vi "Setting.vi"() -> ()   [LabVIEW 2020]
uses:
  Libraries/S7/S7.lvlib
  Global_Variable/Global.vi
  <userlib>/_MGI/1D Array/MGI Average/MGI Average (DBL[]).vi
panel:
  in  "速度":sgl format="%#_3f RMP"
  out "退出":bool=TRUE
  in  "STEP":string
  in  "工位二标定":bool
  in  "停止":bool
  in  "工位一标定":bool
  out "标定曲线":cluster{dbl[], dbl[]}[](graph)
  # "配置标定"
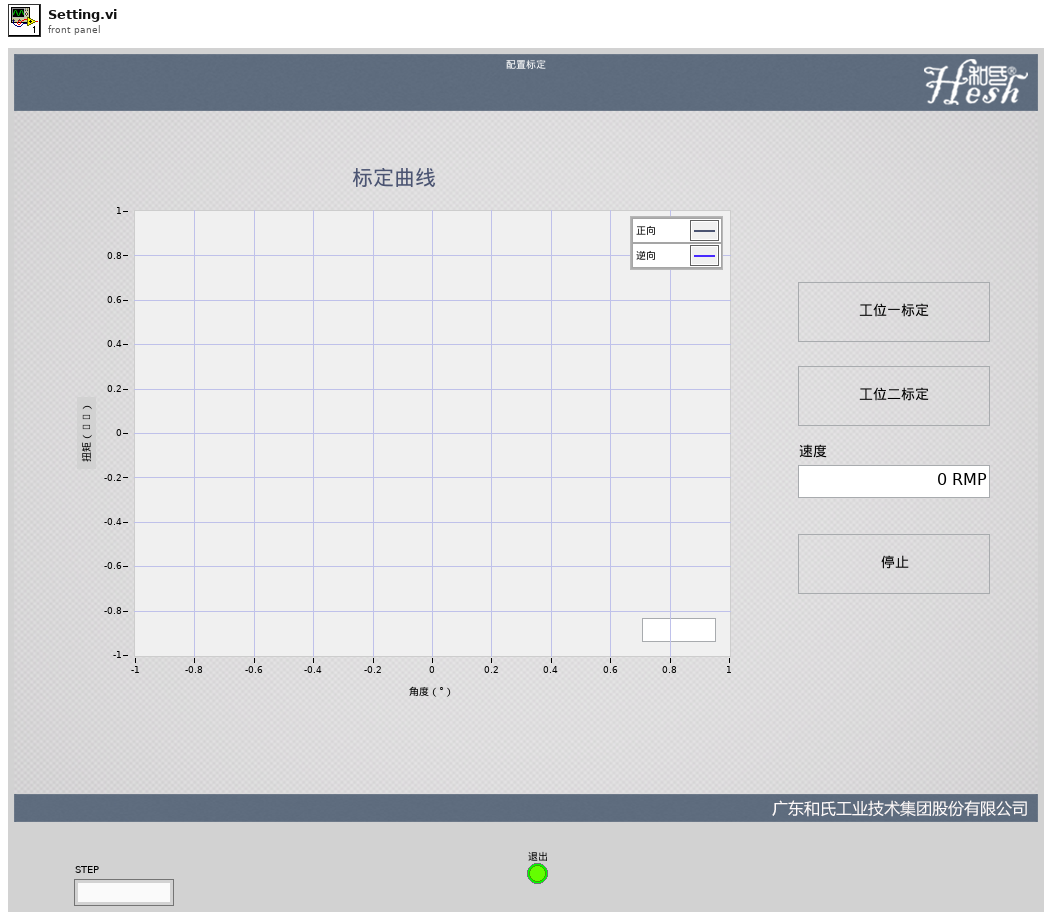
[diagram p1: front panel]
types:
  T1 = cluster{"左工位驱动伺服位移":sgl, "右工位驱动伺服位移":sgl, "横向伺服位移":sgl, "左加载伺服位移":sgl, "右加载伺服位移":sgl}
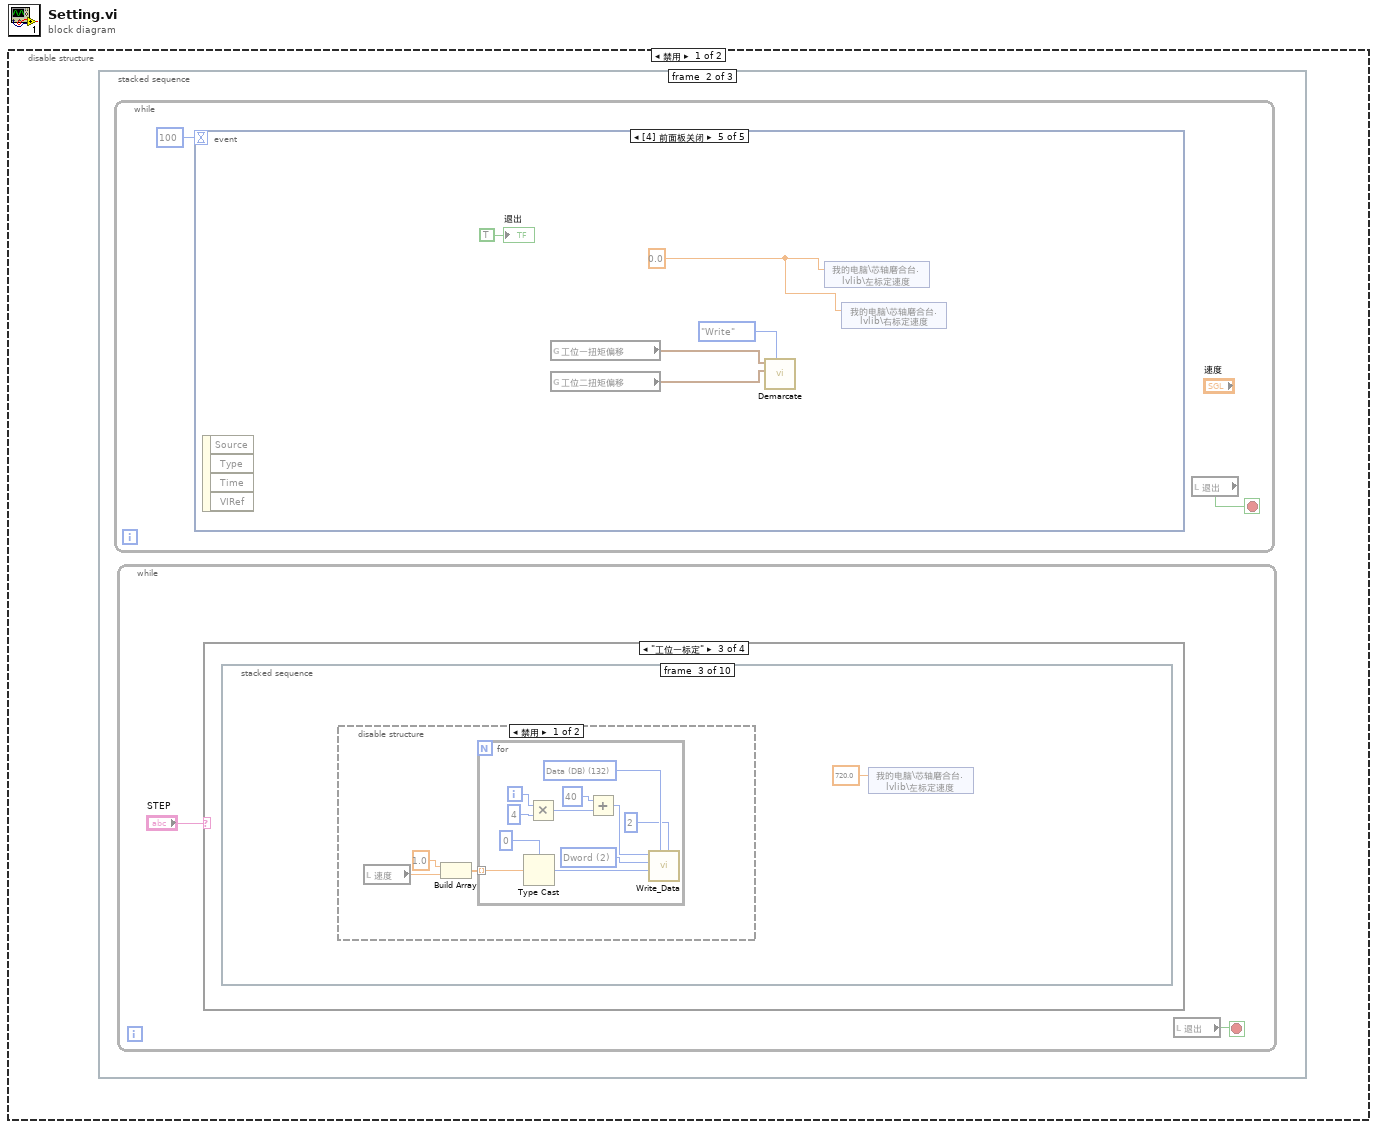
[diagram p0: block diagram]
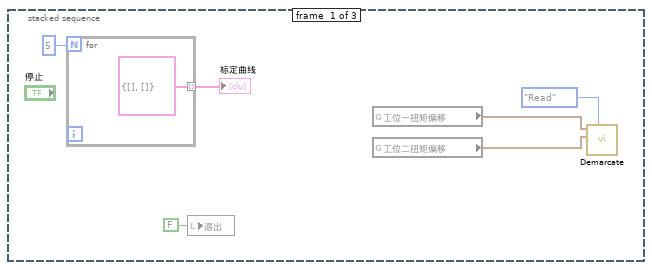
[diagram p2: hidden frame]
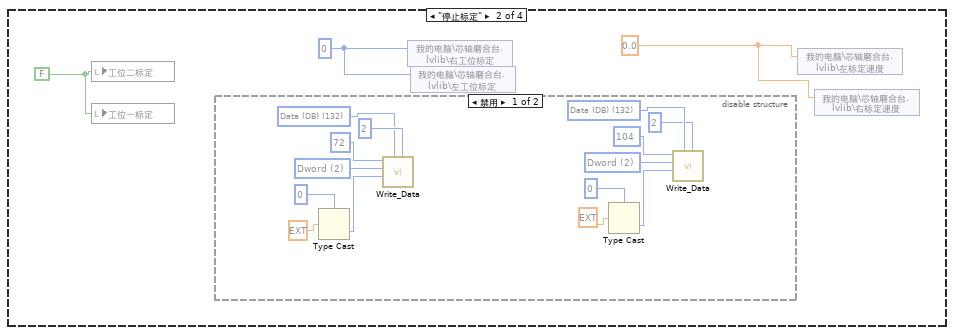
[diagram p4: hidden frame]
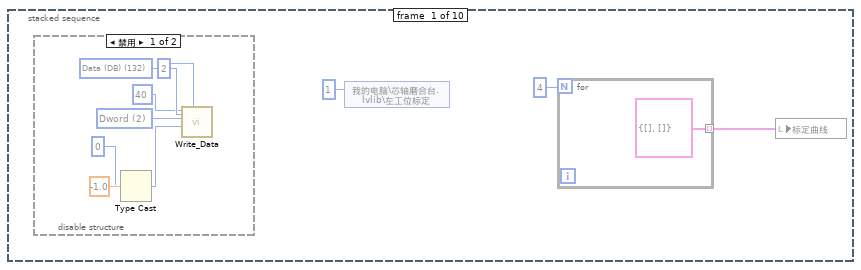
[diagram p6: hidden frame]
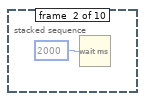
[diagram p8: hidden frame]
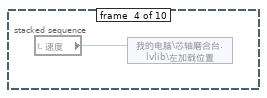
[diagram p10: hidden frame]
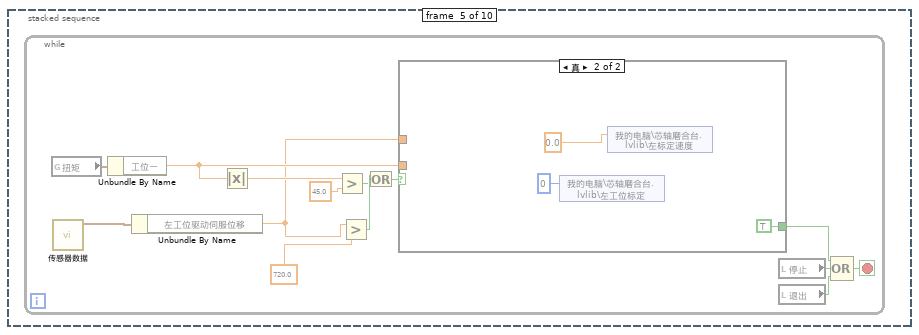
[diagram p11: hidden frame]
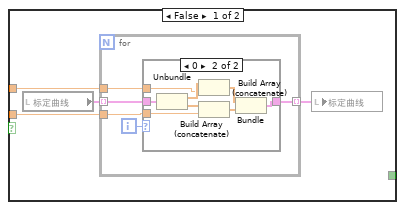
[diagram p12: hidden frame]
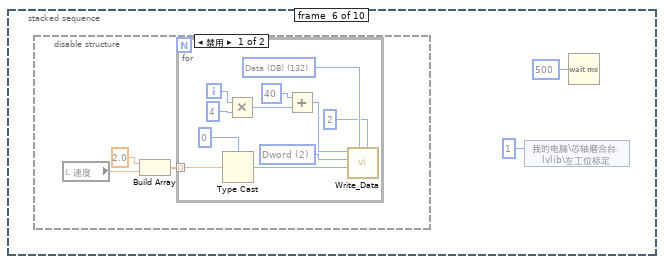
[diagram p14: hidden frame]
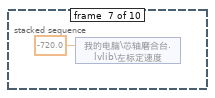
[diagram p16: hidden frame]
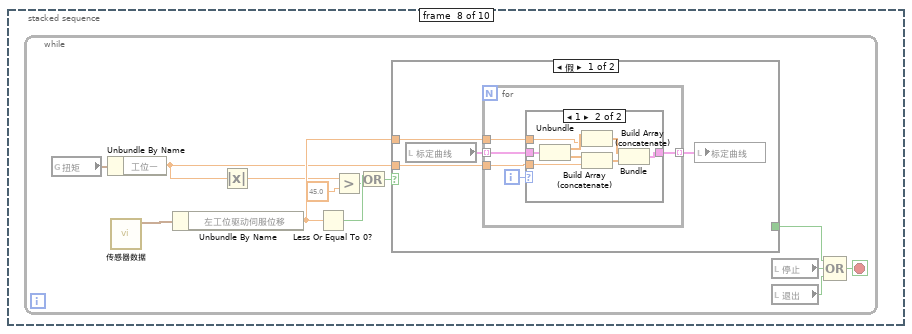
[diagram p17: hidden frame]
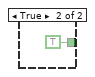
[diagram p19: hidden frame]
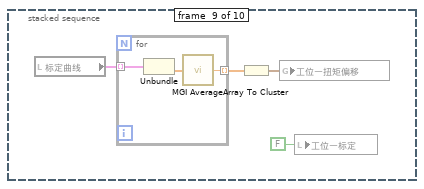
[diagram p20: hidden frame]
diagram:
  n1 = disable-structure shown="禁用" {
    frame Disabled {
      n2 = stacked-sequence {
        frame #0 {
          n3 = for {
            N: 5 -> [_]
            tunnel: [cluster{dbl[], dbl[]} {[], []}] -> w5 mode=indexing
          }
          "标定曲线" <- w5
          n4 = local write "退出"(FALSE ("退出")) -> ()
          n5 = global read "Global.vi" "工位一扭矩偏移"() -> (w3:cluster{"正向":dbl, "逆向":dbl})
          n6 = global read "Global.vi" "工位二扭矩偏移"() -> (w2:cluster{"正向":dbl, "逆向":dbl})
          n7 = call "Demarcate.vi"("Mode"=enum16{"Read", "Write"}."Read", "工位二扭矩偏移"=w2, "工位一扭矩偏移"=w3) -> ()  [unwired: 7 in, 2 out]
        }
        frame #1 {
          n8 = while {
            stop <- w239 stop-if-true
            n9 = event shown="[4] 前面板关闭" {
              selector: _ -> [_ _ _ _ _]
              dyn-events: _ -> [_ _ _ _ _]
              timeout: 100 -> [_ _ _ _ _]
              event Timeout {
                n10 = event-data() -> ()  [unwired: 1 in, 3 out]
              }
              event "工位一标定": Value Change {
                n11 = event-data() -> ()  [unwired: 1 in, 4 out]
                n12 = local write "STEP"("工位一标定" ("STEP")) -> ()
              }
              event "停止": Value Change {
                n13 = event-data() -> ()  [unwired: 1 in, 4 out]
                n14 = local write "STEP"("停止标定" ("STEP")) -> ()
              }
              event "工位二标定": Value Change {
                n15 = event-data() -> ()  [unwired: 1 in, 4 out]
                n16 = local write "STEP"("工位二标定" ("STEP")) -> ()
              }
              event Panel Close {
                w244 = sgl 0.0 ("空载速度")
                n17 = event-data() -> ()  [unwired: 1 in, 4 out]
                n18 = global read "Global.vi" "工位一扭矩偏移"() -> (w246:cluster{"正向":dbl, "逆向":dbl})
                n19 = global read "Global.vi" "工位二扭矩偏移"() -> (w245:cluster{"正向":dbl, "逆向":dbl})
                n20 = call "Demarcate.vi"("Mode"=enum16{"Read", "Write"}."Write", "工位二扭矩偏移"=w245, "工位一扭矩偏移"=w246) -> ()  [unwired: 7 in, 2 out]
                n21 = shared-variable "我的电脑\\芯轴磨合台.lvlib\\左标定速度"(w244) -> ()  [unwired: 1 in, 1 out]
                n22 = shared-variable "我的电脑\\芯轴磨合台.lvlib\\右标定速度"(w244) -> ()  [unwired: 1 in, 1 out]
                "退出" <- TRUE ("退出")
              }
            }
            n23 = local read "退出"() -> (w239:bool)
          }
          n24 = while {
            stop <- w8 stop-if-true
            n25 = case shown="\"工位一标定\"" "STEP" {
              frame "假", Default {
              }
              frame "停止标定" {
                w10 = FALSE ("工位二标定")
                w12 = u16 0 ("右工位标定")
                w11 = sgl 0.0 ("空载速度")
                n26 = local write "工位二标定"(w10) -> ()
                n27 = local write "工位一标定"(w10) -> ()
                n28 = disable-structure shown="禁用" {
                  frame Disabled {
                    w16 = u16 2 items=["byte", "word", "Dword"] ("数据类型")
                    w18 = u8 132 items=["I/O (P)"=128, "Input (I)"=129, "Output (Q)"=130, "Bit Memory (M)"=131, "Data (DB)"=132, "Instance Data (DI)"=133, "Local Data (L)"=134, "Predecessor Local Data (VL)"=135] ("寄存器类型")
                    w23 = u16 2 items=["byte", "word", "Dword"] ("数据类型")
                    w21 = u8 132 items=["I/O (P)"=128, "Input (I)"=129, "Output (Q)"=130, "Bit Memory (M)"=131, "Data (DB)"=132, "Instance Data (DI)"=133, "Local Data (L)"=134, "Predecessor Local Data (VL)"=135] ("寄存器类型")
                    n29 = Type Cast(type=u32 0, x=ext 0.0) -> (*(type *) &x=w25:u32)
                    n30 = call "Write_Data.vi"("DB #"=u16 2, "寄存器类型"=w21, "写入数据"=w25, "数据类型"=w23, "写入地址"=u32 72) -> ()  [unwired: 4 in, 3 out]
                    n31 = Type Cast(type=u32 0, x=ext 0.0) -> (*(type *) &x=w14:u32)
                    n32 = call "Write_Data.vi"("DB #"=u16 2, "寄存器类型"=w18, "写入数据"=w14, "数据类型"=w16, "写入地址"=u32 104) -> ()  [unwired: 4 in, 3 out]
                  }
                  frame Enabled {
                  }
                }
                n33 = shared-variable "我的电脑\\芯轴磨合台.lvlib\\右工位标定"(w12) -> ()  [unwired: 1 in, 1 out]
                n34 = shared-variable "我的电脑\\芯轴磨合台.lvlib\\左工位标定"(w12) -> ()  [unwired: 1 in, 1 out]
                n35 = shared-variable "我的电脑\\芯轴磨合台.lvlib\\左标定速度"(w11) -> ()  [unwired: 1 in, 1 out]
                n36 = shared-variable "我的电脑\\芯轴磨合台.lvlib\\右标定速度"(w11) -> ()  [unwired: 1 in, 1 out]
              }
              frame "工位一标定" {
                n37 = stacked-sequence {
                  frame #0 {
                    n38 = disable-structure shown="禁用" {
                      frame Disabled {
                        w33 = u16 2 items=["byte", "word", "Dword"] ("数据类型")
                        w35 = u8 132 items=["I/O (P)"=128, "Input (I)"=129, "Output (Q)"=130, "Bit Memory (M)"=131, "Data (DB)"=132, "Instance Data (DI)"=133, "Local Data (L)"=134, "Predecessor Local Data (VL)"=135] ("寄存器类型")
                        n39 = Type Cast(type=u32 0, x=sgl -1.0 ("元素")) -> (*(type *) &x=w31:u32)
                        n40 = call "Write_Data.vi"("DB #"=u16 2, "寄存器类型"=w35, "写入数据"=w31, "数据类型"=w33, "写入地址"=u32 40) -> ()  [unwired: 4 in, 3 out]
                      }
                      frame Enabled {
                      }
                    }
                    n41 = shared-variable "我的电脑\\芯轴磨合台.lvlib\\左工位标定"(u16 1 ("左工位标定")) -> ()  [unwired: 1 in, 1 out]
                    n42 = for {
                      N: 4 -> [_]
                      tunnel: [cluster{dbl[], dbl[]} {[], []}] -> w29 mode=indexing
                    }
                    n43 = local write "标定曲线"(w29) -> ()
                  }
                  frame #1 {
                    n44 = Wait (ms)(milliseconds to wait=u32 2000 ("等待时间（毫秒）")) -> ()  [unwired: 1 out]
                  }
                  frame #2 {
                    n45 = disable-structure shown="禁用" {
                      frame Disabled {
                        n46 = local read "速度"() -> (w40:sgl)
                        n47 = Build Array(sgl 1.0 ("元素"), w40) -> (w41:sgl[])
                        n48 = for {
                          tunnel: w41 -> [w48] mode=indexing
                          i -> [w45]
                          w50 = u16 2 items=["byte", "word", "Dword"] ("数据类型")
                          w53 = u8 132 items=["I/O (P)"=128, "Input (I)"=129, "Output (Q)"=130, "Bit Memory (M)"=131, "Data (DB)"=132, "Instance Data (DI)"=133, "Local Data (L)"=134, "Predecessor Local Data (VL)"=135] ("寄存器类型")
                          n49 = Type Cast(type=u32 0, x=w48) -> (*(type *) &x=w47:u32)
                          n50 = Multiply(x=w45, y=u32 4) -> (x*y=w44:u32)
                          n51 = Add(x=u32 40 ("写入地址"), y=w44) -> (x+y=w43:u32)
                          n52 = call "Write_Data.vi"("DB #"=u16 2, "寄存器类型"=w53, "写入数据"=w47, "数据类型"=w50, "写入地址"=w43) -> ()  [unwired: 4 in, 3 out]
                        }
                      }
                      frame Enabled {
                      }
                    }
                    n53 = shared-variable "我的电脑\\芯轴磨合台.lvlib\\左标定速度"(sgl 720.0 ("左标定速度")) -> ()  [unwired: 1 in, 1 out]
                  }
                  frame #3 {
                    n54 = local read "速度"() -> (w54:sgl)
                    n55 = shared-variable "我的电脑\\芯轴磨合台.lvlib\\左加载位置"(w54) -> ()  [unwired: 1 in, 1 out]
                  }
                  frame #4 {
                    n56 = while {
                      stop <- w67 stop-if-true
                      n57 = global read "Global.vi" "扭矩"() -> (w64:cluster{"工位一":dbl, "工位二":dbl})
                      n58 = call "传感器数据.vi"() -> ("传感器读数"=w68:T1)  [unwired: 11 in]
                      n59 = Unbundle By Name(w64) -> ("工位一"=w58:dbl)
                      n60 = Unbundle By Name(w68) -> ("左工位驱动伺服位移"=w56:sgl)
                      n61 = Absolute Value(x=w58) -> (abs(x)=w63:dbl)
                      n62 = Greater?(x=w63, y=45.0) -> (0:w60:bool)
                      n63 = Greater?(x=w56, y=sgl 720.0) -> (0:w61:bool)
                      n64 = Or(x=w61, y=w60) -> (x .or. y?=w59:bool)
                      n65 = case shown="真" w59 {
                        tunnel: [_ TRUE] -> w66
                        tunnel: w56 -> [w71 _]
                        tunnel: w58 -> [w70 _]
                        frame False {
                          n66 = local read "标定曲线"() -> (w72:cluster{dbl[], dbl[]}[])
                          n67 = for {
                            tunnel: w72 -> [w77] mode=indexing
                            tunnel: w71 -> [w76]
                            tunnel: w70 -> [w75]
                            tunnel: [w73] -> w69 mode=indexing
                            i -> [w74]
                            n68 = case shown="0" w74 {
                              tunnel: w77 -> [w78 w86]
                              tunnel: w76 -> [_ w83]
                              tunnel: w75 -> [_ w82]
                              tunnel: [w78 w79] -> w73
                              frame Default {
                              }
                              frame 0 {
                                n69 = Unbundle(w86) -> (w84:dbl[], w85:dbl[])
                                n70 = Build Array (concatenate)(w84, w83) -> (w81:dbl[])
                                n71 = Build Array (concatenate)(w85, w82) -> (w80:dbl[])
                                n72 = Bundle(w81, w80) -> (w79:cluster{dbl[], dbl[]})  [unwired: 1 in]
                              }
                            }
                          }
                          n73 = local write "标定曲线"(w69) -> ()
                        }
                        frame True {
                          n74 = shared-variable "我的电脑\\芯轴磨合台.lvlib\\左工位标定"(u16 0 ("左工位标定")) -> ()  [unwired: 1 in, 1 out]
                          n75 = shared-variable "我的电脑\\芯轴磨合台.lvlib\\左标定速度"(sgl 0.0 ("空载速度")) -> ()  [unwired: 1 in, 1 out]
                        }
                      }
                      n76 = local read "停止"() -> (w65:bool)
                      n77 = local read "退出"() -> (w57:bool)
                      n78 = Compound Arithmetic op=OR ("复合运算")(w66, w65, w57) -> (w67:bool)
                    }
                  }
                  frame #5 {
                    n79 = disable-structure shown="禁用" {
                      frame Disabled {
                        n80 = local read "速度"() -> (w92:sgl)
                        n81 = Build Array(sgl 2.0 ("元素"), w92) -> (w93:sgl[])
                        n82 = for {
                          tunnel: w93 -> [w100] mode=indexing
                          i -> [w97]
                          w102 = u16 2 items=["byte", "word", "Dword"] ("数据类型")
                          w105 = u8 132 items=["I/O (P)"=128, "Input (I)"=129, "Output (Q)"=130, "Bit Memory (M)"=131, "Data (DB)"=132, "Instance Data (DI)"=133, "Local Data (L)"=134, "Predecessor Local Data (VL)"=135] ("寄存器类型")
                          n83 = Type Cast(type=u32 0, x=w100) -> (*(type *) &x=w99:u32)
                          n84 = Multiply(x=w97, y=u32 4) -> (x*y=w96:u32)
                          n85 = Add(x=u32 40 ("写入地址"), y=w96) -> (x+y=w95:u32)
                          n86 = call "Write_Data.vi"("DB #"=u16 2, "寄存器类型"=w105, "写入数据"=w99, "数据类型"=w102, "写入地址"=w95) -> ()  [unwired: 4 in, 3 out]
                        }
                      }
                      frame Enabled {
                      }
                    }
                    n87 = shared-variable "我的电脑\\芯轴磨合台.lvlib\\左工位标定"(u16 1 ("左工位标定")) -> ()  [unwired: 1 in, 1 out]
                    n88 = Wait (ms)(milliseconds to wait=u32 500 ("等待时间（毫秒）")) -> ()  [unwired: 1 out]
                  }
                  frame #6 {
                    n89 = shared-variable "我的电脑\\芯轴磨合台.lvlib\\左标定速度"(sgl -720.0 ("左标定速度")) -> ()  [unwired: 1 in, 1 out]
                  }
                  frame #7 {
                    n90 = while {
                      stop <- w118 stop-if-true
                      n91 = global read "Global.vi" "扭矩"() -> (w114:cluster{"工位一":dbl, "工位二":dbl})
                      n92 = Unbundle By Name(w114) -> ("工位一"=w108:dbl)
                      n93 = call "传感器数据.vi"() -> ("传感器读数"=w119:T1)  [unwired: 11 in]
                      n94 = Unbundle By Name(w119) -> ("左工位驱动伺服位移"=w115:sgl)
                      n95 = Absolute Value(x=w108) -> (abs(x)=w113:dbl)
                      n96 = Less Or Equal To 0?(x=w115) -> (x <= 0?=w111:bool)
                      n97 = Greater?(x=w113, y=45.0) -> (0:w110:bool)
                      n98 = Or(x=w111, y=w110) -> (x .or. y?=w109:bool)
                      n99 = case shown="假" w109 {
                        tunnel: [_ TRUE] -> w117
                        tunnel: w115 -> [w122 _]
                        tunnel: w108 -> [w121 _]
                        frame False {
                          n100 = local read "标定曲线"() -> (w123:cluster{dbl[], dbl[]}[])
                          n101 = for {
                            tunnel: w123 -> [w128] mode=indexing
                            tunnel: w122 -> [w127]
                            tunnel: w121 -> [w126]
                            tunnel: [w124] -> w120 mode=indexing
                            i -> [w125]
                            n102 = case shown="1" w125 {
                              tunnel: w128 -> [w129 w137]
                              tunnel: w127 -> [_ w134]
                              tunnel: w126 -> [_ w133]
                              tunnel: [w129 w130] -> w124
                              frame Default {
                              }
                              frame 1 {
                                n103 = Unbundle(w137) -> (w135:dbl[], w136:dbl[])
                                n104 = Build Array (concatenate)(w135, w134) -> (w132:dbl[])
                                n105 = Build Array (concatenate)(w136, w133) -> (w131:dbl[])
                                n106 = Bundle(w132, w131) -> (w130:cluster{dbl[], dbl[]})  [unwired: 1 in]
                              }
                            }
                          }
                          n107 = local write "标定曲线"(w120) -> ()
                        }
                        frame True {
                        }
                      }
                      n108 = local read "停止"() -> (w116:bool)
                      n109 = local read "退出"() -> (w107:bool)
                      n110 = Compound Arithmetic op=OR ("复合运算")(w117, w116, w107) -> (w118:bool)
                    }
                  }
                  frame #8 {
                    n111 = local read "标定曲线"() -> (w142:cluster{dbl[], dbl[]}[])
                    n112 = for {
                      tunnel: w142 -> [w145] mode=indexing
                      tunnel: [w143] -> w141 mode=indexing
                      n113 = Unbundle(w145) -> (w144:dbl[])  [unwired: 1 out]
                      n114 = call-poly <userlib>:"MGI Average.vi"("Double[]"=w144) -> ("Average"=w143:dbl)  [unwired: 1 in]
                    }
                    n115 = Array To Cluster(array=w141) -> (cluster=w140:cluster{"[0]":dbl, "[1]":dbl})
                    n116 = global write "Global.vi" "工位一扭矩偏移"(w140) -> ()
                    n117 = local write "工位一标定"(FALSE ("工位一标定")) -> ()
                  }
                  frame #9 {
                    w146 = sgl 0.0 ("空载速度")
                    n118 = shared-variable "我的电脑\\芯轴磨合台.lvlib\\左工位标定"(w146) -> ()  [unwired: 1 in, 1 out]
                    n119 = shared-variable "我的电脑\\芯轴磨合台.lvlib\\左标定速度"(w146) -> ()  [unwired: 1 in, 1 out]
                  }
                }
              }
              frame "工位二标定" {
                n120 = stacked-sequence {
                  frame #0 {
                    n121 = disable-structure shown="禁用" {
                      frame Disabled {
                        w153 = u16 2 items=["byte", "word", "Dword"] ("数据类型")
                        w155 = u8 132 items=["I/O (P)"=128, "Input (I)"=129, "Output (Q)"=130, "Bit Memory (M)"=131, "Data (DB)"=132, "Instance Data (DI)"=133, "Local Data (L)"=134, "Predecessor Local Data (VL)"=135] ("寄存器类型")
                        n122 = Type Cast(type=u32 0, x=sgl -1.0 ("元素")) -> (*(type *) &x=w151:u32)
                        n123 = call "Write_Data.vi"("DB #"=u16 2, "寄存器类型"=w155, "写入数据"=w151, "数据类型"=w153, "写入地址"=u32 56) -> ()  [unwired: 4 in, 3 out]
                      }
                      frame Enabled {
                      }
                    }
                    n124 = shared-variable "我的电脑\\芯轴磨合台.lvlib\\右工位标定"(u16 1 ("右工位标定")) -> ()  [unwired: 1 in, 1 out]
                    n125 = for {
                      N: 4 -> [_]
                      tunnel: [cluster{dbl[], dbl[]} {[], []}] -> w149 mode=indexing
                    }
                    n126 = local write "标定曲线"(w149) -> ()
                  }
                  frame #1 {
                    n127 = Wait (ms)(milliseconds to wait=u32 2000 ("等待时间（毫秒）")) -> ()  [unwired: 1 out]
                  }
                  frame #2 {
                    n128 = local read "速度"() -> (w159:sgl)
                    n129 = shared-variable "我的电脑\\芯轴磨合台.lvlib\\右加载位置"(w159) -> ()  [unwired: 1 in, 1 out]
                  }
                  frame #3 {
                    n130 = shared-variable "我的电脑\\芯轴磨合台.lvlib\\右标定速度"(sgl 720.0 ("右标定速度")) -> ()  [unwired: 1 in, 1 out]
                  }
                  frame #4 {
                    n131 = while {
                      stop <- w174 stop-if-true
                      n132 = global read "Global.vi" "扭矩"() -> (w171:cluster{"工位一":dbl, "工位二":dbl})
                      n133 = call "传感器数据.vi"() -> ("传感器读数"=w161:T1)  [unwired: 11 in]
                      n134 = Unbundle By Name(w171) -> ("工位二"=w165:dbl)
                      n135 = Unbundle By Name(w161) -> ("右工位驱动伺服位移"=w163:sgl)
                      n136 = Absolute Value(x=w165) -> (abs(x)=w170:dbl)
                      n137 = Greater?(x=w170, y=45.0) -> (0:w167:bool)
                      n138 = Greater?(x=w163, y=sgl 720.0) -> (0:w168:bool)
                      n139 = Or(x=w168, y=w167) -> (x .or. y?=w166:bool)
                      n140 = case shown="真" w166 {
                        tunnel: [_ TRUE] -> w173
                        tunnel: w163 -> [w177 _]
                        tunnel: w165 -> [w176 _]
                        frame False {
                          n141 = local read "标定曲线"() -> (w178:cluster{dbl[], dbl[]}[])
                          n142 = for {
                            tunnel: w178 -> [w183] mode=indexing
                            tunnel: w177 -> [w182]
                            tunnel: w176 -> [w181]
                            tunnel: [w179] -> w175 mode=indexing
                            i -> [w180]
                            n143 = case shown="默认" w180 {
                              tunnel: w183 -> [w184 w192]
                              tunnel: w182 -> [_ w189]
                              tunnel: w181 -> [_ w188]
                              tunnel: [w184 w185] -> w179
                              frame Default {
                              }
                              frame 0 {
                                n144 = Unbundle(w192) -> (w190:dbl[], w191:dbl[])
                                n145 = Build Array (concatenate)(w190, w189) -> (w187:dbl[])
                                n146 = Build Array (concatenate)(w191, w188) -> (w186:dbl[])
                                n147 = Bundle(w187, w186) -> (w185:cluster{dbl[], dbl[]})  [unwired: 1 in]
                              }
                            }
                          }
                          n148 = local write "标定曲线"(w175) -> ()
                        }
                        frame True {
                          n149 = shared-variable "我的电脑\\芯轴磨合台.lvlib\\右工位标定"(u16 0 ("右工位标定")) -> ()  [unwired: 1 in, 1 out]
                          n150 = shared-variable "我的电脑\\芯轴磨合台.lvlib\\右标定速度"(sgl 0.0 ("空载速度")) -> ()  [unwired: 1 in, 1 out]
                        }
                      }
                      n151 = local read "停止"() -> (w172:bool)
                      n152 = local read "退出"() -> (w164:bool)
                      n153 = Compound Arithmetic op=OR ("复合运算")(w173, w172, w164) -> (w174:bool)
                    }
                  }
                  frame #5 {
                    n154 = shared-variable "我的电脑\\芯轴磨合台.lvlib\\右工位标定"(u16 1 ("右工位标定")) -> ()  [unwired: 1 in, 1 out]
                    n155 = Wait (ms)(milliseconds to wait=u32 500 ("等待时间（毫秒）")) -> ()  [unwired: 1 out]
                  }
                  frame #6 {
                    n156 = shared-variable "我的电脑\\芯轴磨合台.lvlib\\右标定速度"(sgl 720.0 ("右标定速度")) -> ()  [unwired: 1 in, 1 out]
                  }
                  frame #7 {
                    n157 = while {
                      stop <- w210 stop-if-true
                      n158 = global read "Global.vi" "扭矩"() -> (w206:cluster{"工位一":dbl, "工位二":dbl})
                      n159 = call "传感器数据.vi"() -> ("传感器读数"=w211:T1)  [unwired: 11 in]
                      n160 = Unbundle By Name(w206) -> ("工位二"=w200:dbl)
                      n161 = Unbundle By Name(w211) -> ("右工位驱动伺服位移"=w207:sgl)
                      n162 = Absolute Value(x=w200) -> (abs(x)=w205:dbl)
                      n163 = Less Or Equal To 0?(x=w207) -> (x <= 0?=w203:bool)
                      n164 = Greater?(x=w205, y=45.0) -> (0:w202:bool)
                      n165 = Or(x=w203, y=w202) -> (x .or. y?=w201:bool)
                      n166 = case shown="假" w201 {
                        tunnel: [_ TRUE] -> w209
                        tunnel: w207 -> [w214 _]
                        tunnel: w200 -> [w213 _]
                        frame False {
                          n167 = local read "标定曲线"() -> (w215:cluster{dbl[], dbl[]}[])
                          n168 = for {
                            tunnel: w215 -> [w220] mode=indexing
                            tunnel: w214 -> [w219]
                            tunnel: w213 -> [w218]
                            tunnel: [w216] -> w212 mode=indexing
                            i -> [w217]
                            n169 = case shown="1" w217 {
                              tunnel: w220 -> [w221 w229]
                              tunnel: w219 -> [_ w226]
                              tunnel: w218 -> [_ w225]
                              tunnel: [w221 w222] -> w216
                              frame Default {
                              }
                              frame 1 {
                                n170 = Unbundle(w229) -> (w227:dbl[], w228:dbl[])
                                n171 = Build Array (concatenate)(w227, w226) -> (w224:dbl[])
                                n172 = Build Array (concatenate)(w228, w225) -> (w223:dbl[])
                                n173 = Bundle(w224, w223) -> (w222:cluster{dbl[], dbl[]})  [unwired: 1 in]
                              }
                            }
                          }
                          n174 = local write "标定曲线"(w212) -> ()
                        }
                        frame True {
                        }
                      }
                      n175 = local read "停止"() -> (w208:bool)
                      n176 = local read "退出"() -> (w199:bool)
                      n177 = Compound Arithmetic op=OR ("复合运算")(w209, w208, w199) -> (w210:bool)
                    }
                  }
                  frame #8 {
                    n178 = local read "标定曲线"() -> (w234:cluster{dbl[], dbl[]}[])
                    n179 = for {
                      tunnel: w234 -> [w237] mode=indexing
                      tunnel: [w235] -> w233 mode=indexing
                      n180 = Unbundle(w237) -> (w236:dbl[])  [unwired: 1 out]
                      n181 = call-poly <userlib>:"MGI Average.vi"("Double[]"=w236) -> ("Average"=w235:dbl)  [unwired: 1 in]
                    }
                    n182 = Array To Cluster(array=w233) -> (cluster=w232:cluster{"[0]":dbl, "[1]":dbl})
                    n183 = global write "Global.vi" "工位二扭矩偏移"(w232) -> ()
                    n184 = local write "工位二标定"(FALSE ("工位一标定")) -> ()
                  }
                  frame #9 {
                    w238 = sgl 0.0 ("空载速度")
                    n185 = shared-variable "我的电脑\\芯轴磨合台.lvlib\\右工位标定"(w238) -> ()  [unwired: 1 in, 1 out]
                    n186 = shared-variable "我的电脑\\芯轴磨合台.lvlib\\右标定速度"(w238) -> ()  [unwired: 1 in, 1 out]
                  }
                }
              }
            }
            n187 = local read "退出"() -> (w8:bool)
          }
        }
        frame #2 {
        }
      }
    }
    frame Enabled {
    }
  }
